vi "上位机.vi"() -> ()   [LabVIEW 2016]
uses:
  <vilib>/Utility/file.llb/Read Delimited Spreadsheet (DBL).vi
panel:
  in  "停止按钮":bool
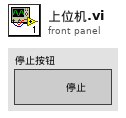
[diagram p1: front panel]
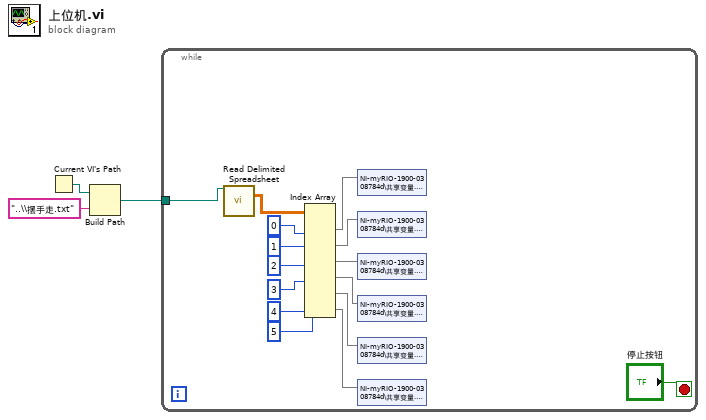
[diagram p0: block diagram]
diagram:
  n1 = Current VI's Path() -> (path=w3:path)
  n2 = Build Path(base path=w3, name or relative path="..\\摆手走.txt" ("名称或相对路径")) -> (appended path=w1:path)
  n3 = while {
    tunnel: w1 -> [w17]
    stop <- "停止按钮" stop-if-true
    n4 = call-poly <vilib>:"Read Delimited Spreadsheet.vi"("file path (dialog if empty)"=w17) -> ("all rows"=w16:dbl[][])  [unwired: 9 in, 5 out]
    n5 = Index Array(array=w16, index (col) #1=0 ("禁用的索引 (列)"), index (col) #2=1 ("索引 (列)"), index (col) #3=2 ("索引 (列)"), index (col) #4=3 ("索引 (列)"), index (col) #5=4 ("索引 (列)"), index (col) #6=5 ("索引 (列)")) -> (element #1=w13:dbl[], element #2=w12:dbl[], element #3=w15:dbl[], element #4=w14:dbl[], element #5=w11:dbl[], element #6=w10:dbl[])  [unwired: 6 in]
    n6 = shared-variable "NI-myRIO-1900-0308784d\\共享变量.lvlib\\左肩"(w13) -> ()  [unwired: 1 in, 1 out]
    n7 = shared-variable "NI-myRIO-1900-0308784d\\共享变量.lvlib\\右肩"(w12) -> ()  [unwired: 1 in, 1 out]
    n8 = shared-variable "NI-myRIO-1900-0308784d\\共享变量.lvlib\\左肘"(w15) -> ()  [unwired: 1 in, 1 out]
    n9 = shared-variable "NI-myRIO-1900-0308784d\\共享变量.lvlib\\右肘"(w14) -> ()  [unwired: 1 in, 1 out]
    n10 = shared-variable "NI-myRIO-1900-0308784d\\共享变量.lvlib\\左手"(w11) -> ()  [unwired: 1 in, 1 out]
    n11 = shared-variable "NI-myRIO-1900-0308784d\\共享变量.lvlib\\右手"(w10) -> ()  [unwired: 1 in, 1 out]
  }
